vi "test VI (1).vi"() -> ()   [LabVIEW 2018]
panel:
  in  "String":string
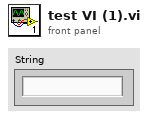
[diagram p1: front panel]
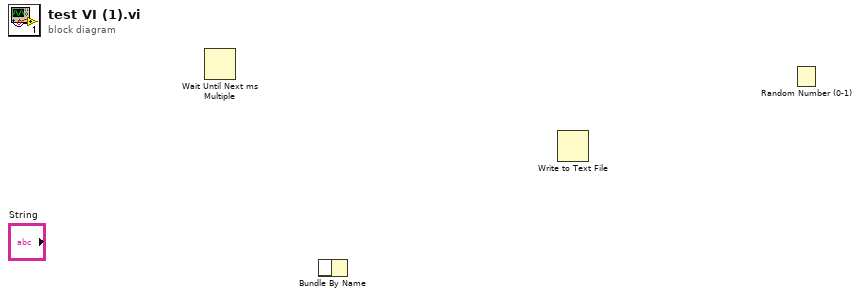
[diagram p0: block diagram]
diagram:
  n1 = Wait Until Next ms Multiple() -> ()  [unwired: 1 in, 1 out]
  n2 = Bundle By Name() -> ()  [unwired: 2 in, 1 out]
  n3 = Write to Text File() -> ()  [unwired: 4 in, 3 out]
  n4 = Random Number (0-1)() -> ()  [unwired: 1 out]
